vi "tabs.vi"() -> ()   [LabVIEW 2015]
panel:
  in  "Measurement type":enum16{""}(ring)
  in  "Cancel Button":bool
  in  "Stop Button":bool
  in  "Record Button":bool
  in  "File Path Control":path
  in  "Tab Control":enum32{"Page 1", "Page 2"}(tab)
  out "Cluster":T1
  out "XY Graph 8":cluster{"X":dbl, "Y":dbl}[](graph)
  out "XY Graph 7":cluster{"X":dbl, "Y":dbl}[](graph)
  out "XY Graph 6":cluster{"X":dbl, "Y":dbl}[](graph)
  out "XY Graph 5":cluster{"X":dbl, "Y":dbl}[](graph)
  out "XY Graph 4":cluster{"X":dbl, "Y":dbl}[](graph)
  out "XY Graph 3":cluster{"X":dbl, "Y":dbl}[](graph)
  out "XY Graph 2":cluster{"X":dbl, "Y":dbl}[](graph)
  out "XY Graph":cluster{"X":dbl, "Y":dbl}[](graph)
  out "Thermometer":dbl(slide) scale=0.0..1000.0
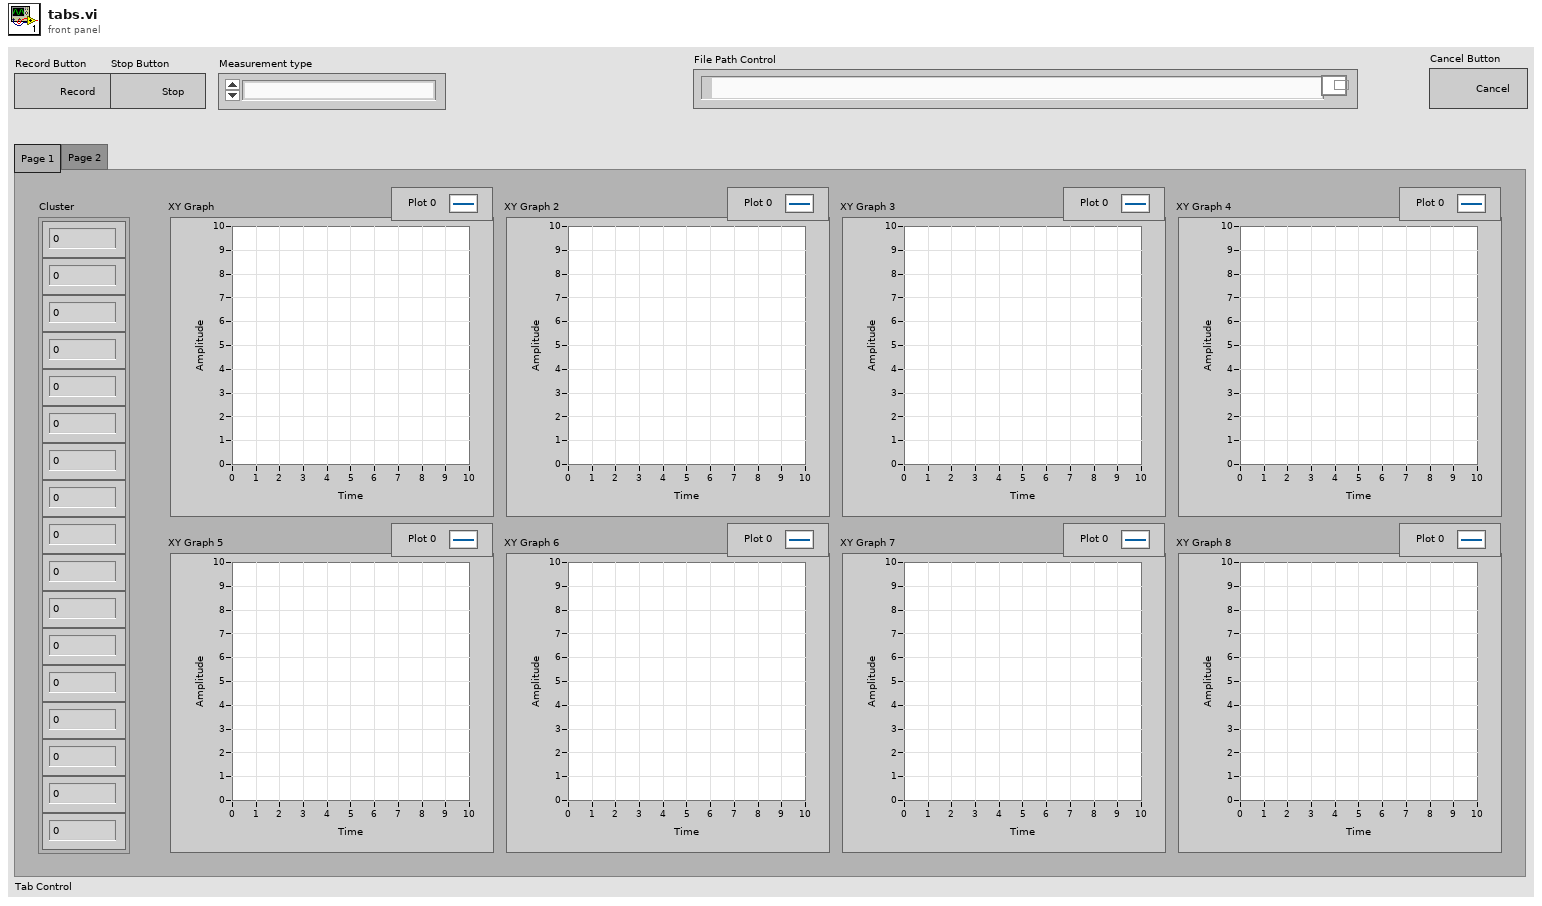
[diagram p1: front panel]
types:
  T1 = cluster{"Numeric Indicator":dbl, "Numeric Indicator 2":dbl, "Numeric Indicator 3":dbl, "Numeric Indicator 4":dbl, "Numeric Indicator 5":dbl, "Numeric Indicator 6":dbl, "Numeric Indicator 7":dbl, "Numeric Indicator 8":dbl, "Numeric Indicator 9":dbl, "Numeric Indicator 10":dbl, "Numeric Indicator 11":dbl, "Numeric Indicator 12":dbl, "Numeric Indicator 13":dbl, "Numeric Indicator 14":dbl, "Numeric Indicator 15":dbl, "Numeric Indicator 16":dbl, "Numeric Indicator 17":dbl}
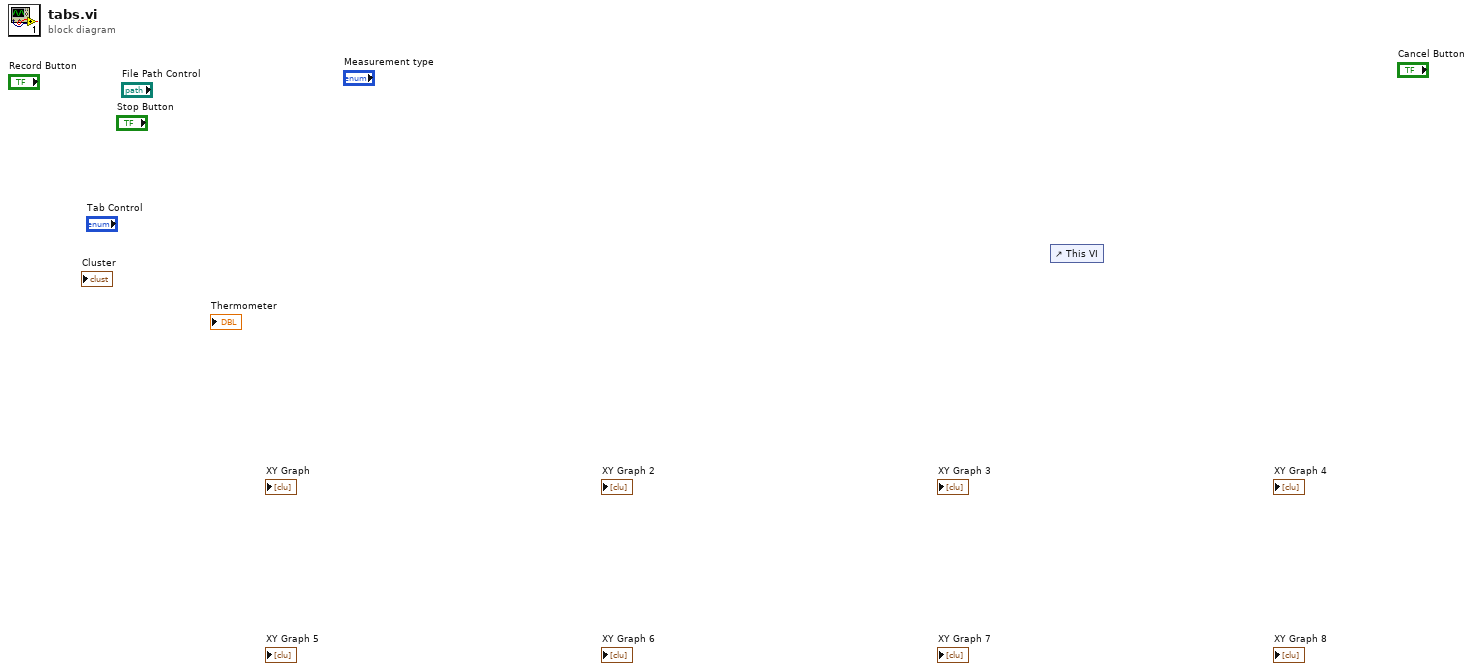
[diagram p0: block diagram]
diagram:
  n1 = control-ref of="This VI"() -> (w1:refnum<vi>)
